vi "Solver_001.vi"(10 "Word List":string[](array[string])=["YELLOW", "ORANGE", "PURPLE", "BLUE", "GREEN", "RED"], 11 "Word Search Grid":string[][](array[string])=[["R", "B", "L", "U", "E", "W"], ["E", "G", "N", "A", "R", "O"], ["D", "B", "C", "E", "W", "L"], ["L", "L", "D", "K", "V", "L"], ["P", "U", "R", "P", "L", "E"], ["N", "E", "E", "R", "G", "Y"]]) -> (3 "Solutions":T1={"BLUE"=[{"Row"=0, "Column"=1}, {"Row"=0, "Column"=2}, {"Row"=0, "Column"=3}, {"Row"=0, "Column"=4}], "GREEN"=[{"Row"=5, "Column"=4}, {"Row"=5, "Column"=3}, {"Row"=5, "Column"=2}, {"Row"=5, "Column"=1}, {"Row"=5, "Column"=0}], "ORANGE"=[{"Row"=1, "Column"=5}, {"Row"=1, "Column"=4}, {"Row"=1, "Column"=3}, {"Row"=1, "Column"=2}, {"Row"=1, "Column"=1}, {"Row"=1, "Column"=0}], "PURPLE"=[{"Row"=4, "Column"=0}, {"Row"=4, "Column"=1}, {"Row"=4, "Column"=2}, {"Row"=4, "Column"=3}, {"Row"=4, "Column"=4}, {"Row"=4, "Column"=5}], "RED"=[{"Row"=0, "Column"=0}, {"Row"=1, "Column"=0}, {"Row"=2, "Column"=0}], "YELLOW"=[{"Row"=5, "Column"=5}, {"Row"=4, "Column"=5}, {"Row"=3, "Column"=5}, {"Row"=2, "Column"=5}, {"Row"=1, "Column"=5}, {"Row"=0, "Column"=5}]})   [LabVIEW 2022 SP3]
uses:
  Solutions--map.ctl
  Letter Index--cluster.ctl
panel:
  # "Do not change the connector pane of this VI."
  # "Observe the default values stored in this VI to understand how each word is represented in the Solutions map.\n\nSee the block diagram for a simple implementation of a solution. Note that this approach is not very efficient, and you will want to come up with a faster way to find the words in the grid."
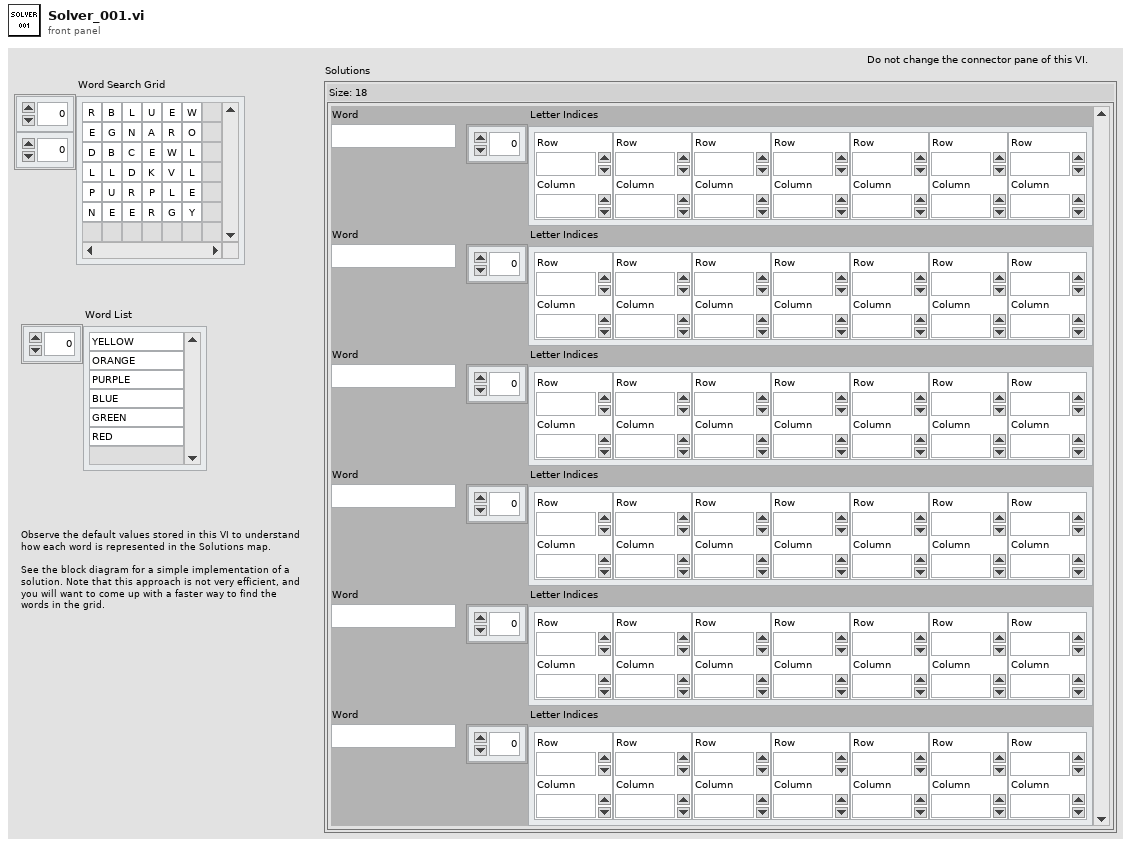
[diagram p1: front panel]
types:
  T1 = typedef "Solutions--map.ctl" = map{string, T2[]}
  T2 = typedef "Letter Index--cluster.ctl" = cluster{"Row":i32, "Column":i32}
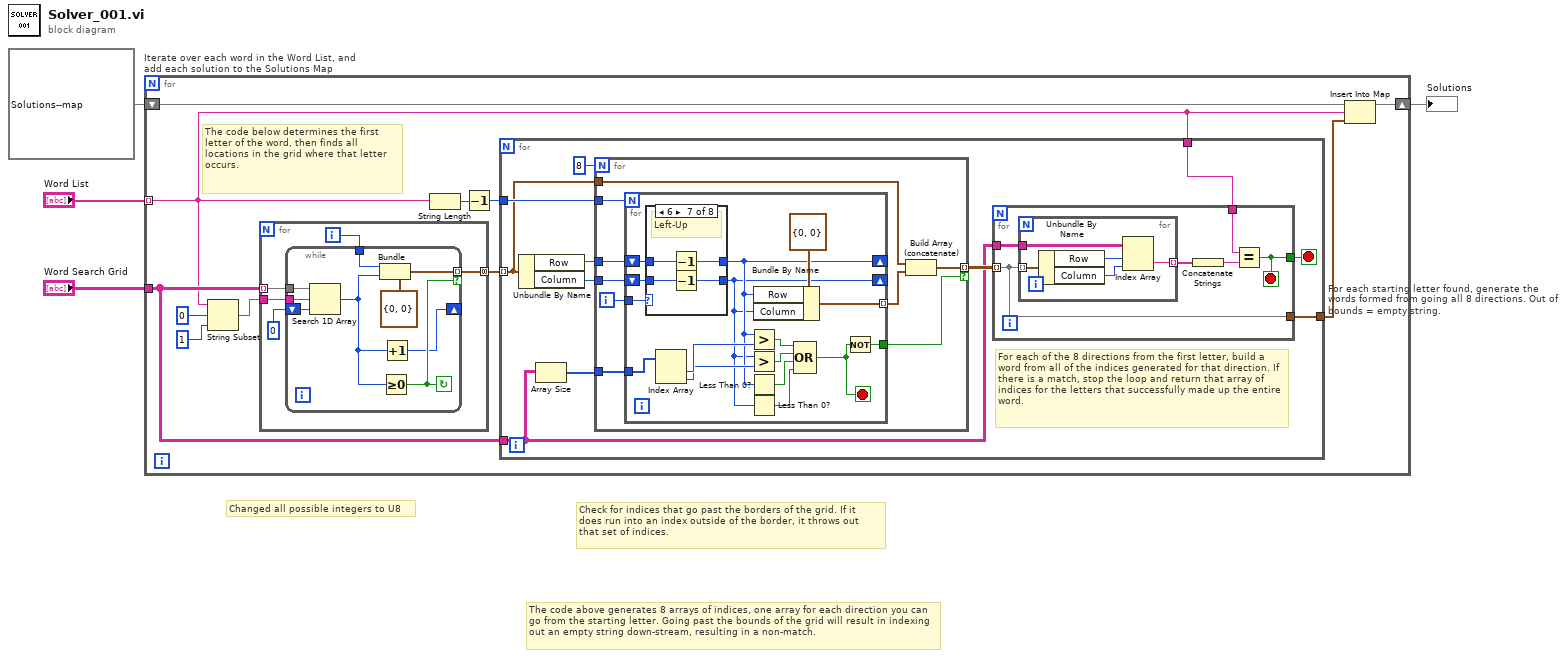
[diagram p0: block diagram]
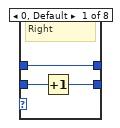
[diagram p2: hidden frame]
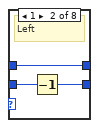
[diagram p3: hidden frame]
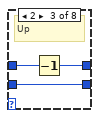
[diagram p4: hidden frame]
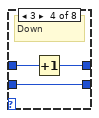
[diagram p5: hidden frame]
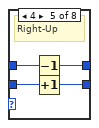
[diagram p6: hidden frame]
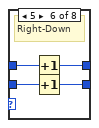
[diagram p7: hidden frame]
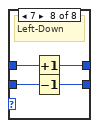
[diagram p8: hidden frame]
diagram:
  # "Check for indices that go past the borders of the grid. If it \ndoes run into an index outside of the border, it throws out\nthat set of indices."
  # "Changed all possible integers to U8"
  # "The code above generates 8 arrays of indices, one array for each direction you can go from the starting letter. Going past the bounds of the grid will result in indexing out an empty string down-stream, resulting in a non-match."
  n1 = for "Iterate over each word in the Word List, and add each solution to the Solutions Map" {
    tunnel: "Word Search Grid" -> [w7]
    tunnel: "Word List" -> [w6] mode=indexing
    shift-right: [w14] -> w4
    shift-left: T1 {} ("Solutions") -> [w15]
    # "The code below determines the first letter of the word, then finds all locations in the grid where that letter occurs."
    n2 = String Subset(string=w6, offset (0)=u8 0, length (rest)=u8 1 ("length (rest)")) -> (substring=w12:string)
    n3 = for {
      tunnel: w7 -> [w95] mode=indexing
      tunnel: w12 -> [w94]
      tunnel: [w92] -> w11 mode=concatenating
      i -> [w93]
      n4 = while {
        tunnel: w95 -> [w104]
        tunnel: w94 -> [w103]
        tunnel: w93 -> [w101]
        tunnel: [w100] -> w92 mode=indexing if=w99
        shift-right: [w96] -> _
        shift-left: 0 -> [w98]
        stop <- w99 continue-if-true
        n5 = Search 1D Array(1D array=w104, element=w103, start index (0)=w98) -> (index of element=w97:i32)
        n6 = Bundle(cluster=T2 {"Row"=0, "Column"=0} ("Letter Index"), "Row"=w101, "Column"=w97) -> (w100:T2)
        n7 = Greater Or Equal To 0?(x=w97) -> (x >= 0?=w99:bool)
        n8 = Increment(x=w97) -> (x+1=w96:i32)
      }
    }
    n9 = String Length(string=w6) -> (length=w9:i32)
    n10 = Decrement(x=w9) -> (x-1=w8:i32)
    n11 = for "For each starting letter found, generate the words formed from going all 8 directions. Out of bounds = empty string." {
      tunnel: w11 -> [w22] mode=indexing
      tunnel: w8 -> [w25]
      tunnel: w7 -> [w17]
      tunnel: [w20] -> w5
      tunnel: w6 -> [w19]
      stop <- w18 stop-if-true
      # "For each of the 8 directions from the first letter, build a word from all of the indices generated for that direction. If there is a match, stop the loop and return that array of indices for the letters that successfully made up the entire word."
      n12 = Unbundle By Name(w22) -> ("Row"=w24:i32, "Column"=w23:i32)
      n13 = Array Size(array=w17) -> (size(s)=w16:i32[])
      n14 = for {
        N: 8 -> [_]
        tunnel: w25 -> [w46]
        tunnel: w24 -> [w45]
        tunnel: w23 -> [w44]
        tunnel: w22 -> [w41]
        tunnel: [w40] -> w21 mode=indexing if=w38
        tunnel: w16 -> [w39]
        i -> [w43]
        n15 = for {
          N: w46 -> [_]
          tunnel: w43 -> [w60]
          tunnel: [w58] -> w42 mode=indexing
          shift-right: [w48] -> _
          shift-left: w45 -> [w62]
          shift-right: [w47] -> _
          shift-left: w44 -> [w61]
          tunnel: w39 -> [w57]
          tunnel: [w51] -> w38
          stop <- w52 stop-if-true
          n16 = case shown="6" w60 {
            tunnel: w62 -> [w63 w66 w70 w73 w77 w81 w85 w89]
            tunnel: w61 -> [w65 w68 w71 w74 w78 w82 w86 w90]
            tunnel: [w64 w67 w71 w74 w75 w79 w83 w87] -> w47
            tunnel: [w63 w66 w69 w72 w76 w80 w84 w88] -> w48
            frame 0, Default {
              # "Right"
              n17 = Increment(x=w65) -> (x+1=w64:i32)
            }
            frame 1 {
              # "Left"
              n18 = Decrement(x=w68) -> (x-1=w67:i32)
            }
            frame 2 {
              # "Up"
              n19 = Decrement(x=w70) -> (x-1=w69:i32)
            }
            frame 3 {
              # "Down"
              n20 = Increment(x=w73) -> (x+1=w72:i32)
            }
            frame 4 {
              # "Right-Up"
              n21 = Decrement(x=w77) -> (x-1=w76:i32)
              n22 = Increment(x=w78) -> (x+1=w75:i32)
            }
            frame 5 {
              # "Right-Down"
              n23 = Increment(x=w81) -> (x+1=w80:i32)
              n24 = Increment(x=w82) -> (x+1=w79:i32)
            }
            frame 6 {
              # "Left-Up"
              n25 = Decrement(x=w85) -> (x-1=w84:i32)
              n26 = Decrement(x=w86) -> (x-1=w83:i32)
            }
            frame 7 {
              # "Left-Down"
              n27 = Increment(x=w89) -> (x+1=w88:i32)
              n28 = Decrement(x=w90) -> (x-1=w87:i32)
            }
          }
          n29 = Index Array(array=w57) -> (element #1=w56:i32, element #2=w55:i32)  [unwired: 2 in]
          n30 = Greater?(x=w48, y=w56) -> (0:w54:bool)
          n31 = Greater?(x=w47, y=w55) -> (0:w53:bool)
          n32 = Less Than 0?(x=w48) -> (x < 0?=w50:bool)
          n33 = Less Than 0?(x=w47) -> (x < 0?=w49:bool)
          n34 = Bundle By Name(cluster=T2 {"Row"=0, "Column"=0} ("Letter Index"), "Row"=w48, "Column"=w47) -> (w58:T2)
          n35 = Compound Arithmetic op=OR(w54, w53, w50, w49) -> (w52:bool)
          n36 = Not(x=w52) -> (.not. x?=w51:bool)
        }
        n37 = Build Array (concatenate)(w41, w42) -> (w40:T2[])
      }
      n38 = for {
        tunnel: w21 -> [w29] mode=indexing
        tunnel: w17 -> [w32]
        tunnel: [w29] -> w20
        tunnel: w19 -> [w28]
        tunnel: [w27] -> w18
        stop <- w27 stop-if-true
        n39 = for {
          tunnel: w29 -> [w37] mode=indexing
          tunnel: w32 -> [w35]
          tunnel: [w33] -> w31 mode=indexing
          n40 = Unbundle By Name(w37) -> ("Row"=w36:i32, "Column"=w34:i32)
          n41 = Index Array(array=w35, index (row)=w36, index (col)=w34) -> (element=w33:string)
        }
        n42 = Concatenate Strings(w31) -> (w30:string)
        n43 = Equal?(x=w28, y=w30) -> (x = y?=w27:bool)
      }
    }
    n44 = Insert Into Map(map in=w15, key=w6, value=w5) -> (map out=w14:T1)  [unwired: 2 out]
  }
  "Solutions" <- w4
